vi "read Output Files.vi"(8 "error in (no error)":errorcluster, 11 "path_to_outputFiles":string) -> (0 "error out":errorcluster, 3 "function return":bool)   [LabVIEW 2019, in "libOutputReader.lvlib"]
doc: "bool readOutputFiles(const char* path_to_outputFiles)"
uses:
  libOutputReader.lvlib
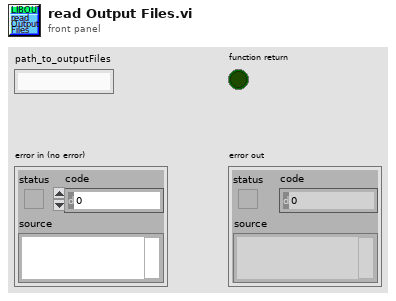
[diagram p1: front panel]
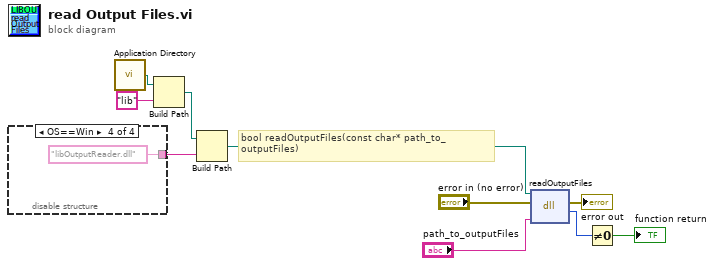
[diagram p0: block diagram]
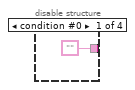
[diagram p2: hidden frame]
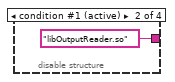
[diagram p3: hidden frame]
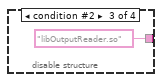
[diagram p4: hidden frame]
diagram:
  # "bool readOutputFiles(const char* path_to_outputFiles)"
  n1 = disable-structure shown="OS==Win" {
    disable-tunnel: ["" "libOutputReader.so" ("name or relative path") "libOutputReader.so" ("name or relative path") "libOutputReader.dll" ("name or relative path")] -> w2
    frame condition #0 {
    }
    frame condition #1 (active) {
    }
    frame condition #2 {
    }
    frame condition #3 {
    }
  }
  n2 = call <vilib>:"Application Directory.vi"() -> ("Application Directory"=w5:path)
  n3 = Build Path(base path=w5, name or relative path="lib") -> (appended path=w3:path)
  n4 = Build Path(base path=w3, name or relative path=w2) -> (appended path=w1:path)
  n5 = dll-call lib="home/paul/Schreibtisch/Biogas_plant_setup/LabView/lib/libOutputReader/libOutputReader.*" fn="readOutputFiles"(path in=w1, error in="error in (no error)", "path_to_outputFiles"="path_to_outputFiles") -> (error out=→"error out":errorcluster, "return type"=w9:u8)  [unwired: 2 in, 1 out]
  n6 = Not Equal To 0?(x=w9) -> (x != 0?=→"function return":bool)
